vi "openEvent.vi"(8 "error in (no error)":errorcluster, 11 "WinX32Settings in":refnum<class "WinX32Settings.lvclass">) -> (0 "error out":errorcluster, 3 "WinX32Settings out":refnum<class "WinX32Settings.lvclass">)   [LabVIEW 2011, in "Tools.lvlib" / "Settings.lvlib" / "WinX32Settings.lvclass"]
uses:
  WinX32Settings.lvclass
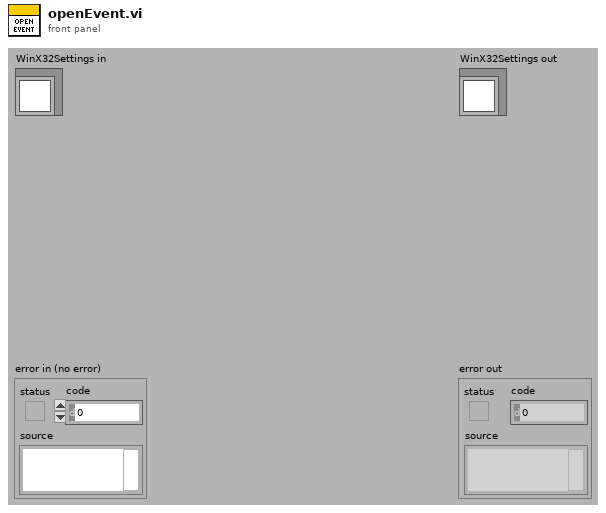
[diagram p1: front panel]
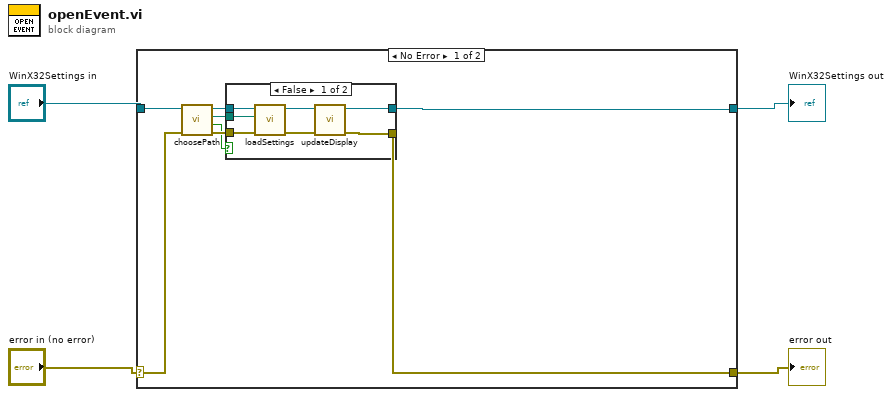
[diagram p0: block diagram]
diagram:
  n1 = case shown="No Error" "error in (no error)" {
    selector: "error in (no error)" -> [w9 w23]
    tunnel: [w12 w23] -> w1
    tunnel: [w8 w22] -> w2
    tunnel: "WinX32Settings in" -> [w10 w22]
    frame No Error {
      n2 = call "choosePath.vi"("error in (no error)"=w9, "WinX32Settings in"=w10) -> ("error out"=w6:errorcluster, "cancelled?"=w5:bool, "Path"=w7:path, "WinX32Settings out"=w11:refnum<class "WinX32Settings.lvclass">)  [unwired: 6 in]
      n3 = case shown="False" w5 {
        tunnel: w11 -> [w19 w20]
        tunnel: w6 -> [w18 w21]
        tunnel: [w15 w21] -> w12
        tunnel: [w14 w20] -> w8
        tunnel: w7 -> [w13 _]
        frame False {
          n4 = call-dynamic "loadSettings.vi"("error in (no error)"=w18, "Path"=w13, "WinX32Settings in"=w19) -> ("error out"=w16:errorcluster, "WinX32Settings out"=w17:refnum<class "WinX32Settings.lvclass">)  [unwired: 7 in]
          n5 = call "updateDisplay.vi"("error in (no error)"=w16, "WinX32Settings in"=w17) -> ("error out"=w15:errorcluster, "WinX32Settings out"=w14:refnum<class "WinX32Settings.lvclass">)  [unwired: 8 in]
        }
        frame True {
        }
      }
    }
    frame Error {
    }
  }
  "error out" <- w1
  "WinX32Settings out" <- w2
